vi "uA_daq_Read_DUT_Voltage.vi"(8 "error in":errorcluster, 11 "USB DAQ":tag) -> (0 "error out":errorcluster, 3 "DUT_Voltage":dbl format="%0.5f")   [LabVIEW 2017]
uses:
  <vilib>/DAQmx/read.llb/DAQmx Read.vi
  <vilib>/DAQmx/read.llb/DAQmx Read (Analog DBL 1Chan 1Samp).vi
  <vilib>/DAQmx/create/channels.llb/DAQmx Create Channel (AI-Voltage-Basic).vi
  <vilib>/DAQmx/miscellaneous.llb/DAQmx Fill In Error Info.vi
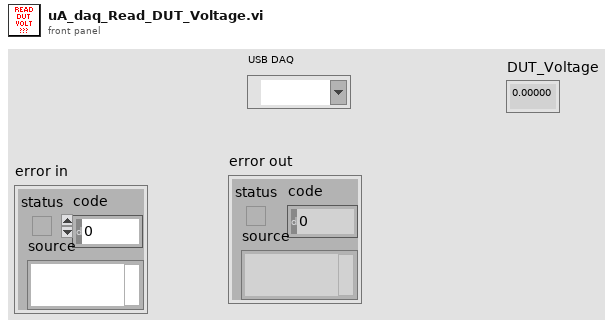
[diagram p1: front panel]
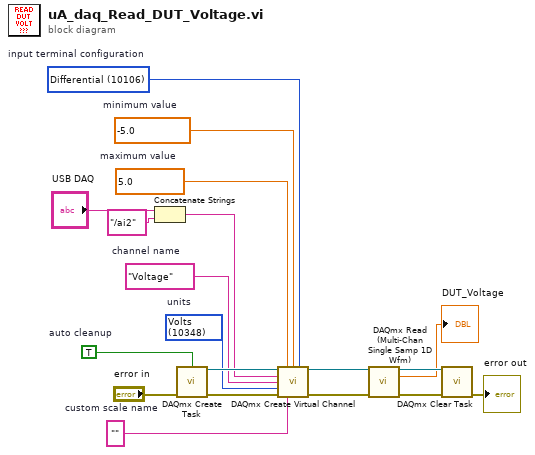
[diagram p0: block diagram]
diagram:
  w8 = 10106 items=["default"=-1, "RSE"=10083, "NRSE"=10078, "Differential"=10106, "Pseudodifferential"=12529]  # input terminal configuration
  w9 = 10348 items=["Volts"=10348, "From Custom Scale"=10065]  # units
  w10 = "Voltage"  # channel name
  w11 = ""  # custom scale name
  w12 = -5.0  # minimum value
  w13 = 5.0  # maximum value
  w15 = TRUE  # auto cleanup
  n1 = Concatenate Strings("USB DAQ", "/ai2" ("string")) -> (w1:string)
  n2 = call <vilib>:"DAQmx Create Task.vi"("auto cleanup"=w15, "error in"="error in") -> ("task out"=w14:refnum<k21>, "error out"=w16:errorcluster)  [unwired: 12 in]
  n3 = call-poly <vilib>:"DAQmx Create Virtual Channel.vi"("task in"=w14, "maximum value"=w13, "minimum value"=w12, "input terminal configuration"=w8, "physical channels"=w1, "name to assign"=w10, "units"=w9, "error in"=w16, "custom scale name"=w11) -> ("task out"=w7:refnum<k21>, "error out"=w6:errorcluster)  [unwired: 5 in]
  n4 = call-poly "DAQmx Read (Multi-Chan Single Samp 1D Wfm).vi"("task/channels in"=w7, "error in"=w6) -> ("task out"=w18:refnum<k21>, "data"=→"DUT_Voltage":dbl, "error out"=w19:errorcluster)  [unwired: 11 in]
  n5 = call <vilib>:"DAQmx Clear Task.vi"("task in"=w18, "error in"=w19) -> ("error out"=→"error out":errorcluster)  [unwired: 13 in]
